vi "SSL Detection Frame Simple Estimator Cameras VelCmd.vi"(0 "Lado":enum16{"Esquerdo", "Direito"}(ring)=enum."Direito" caption="Enum", 4 "Last IA State":T5={"our_robots"=[], "enemy_robots"=[], "balls"=[], "geometry"={"line_width"=0, "field_length"=0, "field_width"=0, "boundary_width"=0, "referee_width"=0, "goal_width"=0, "goal_depth"=0, "goal_wall_width"=0, "center_circle_radius"=0, "defense_radius"=0, "defense_stretch"=0, "free_kick_from_defense_dist"=0, "penalty_spot_from_field_line_dist"=0, "penalty_line_from_spot_dist"=0}, "IA Judge"={"stage"="", "command"="", "our_goalie_id"=0.0, "enemy_goalie_id"=0.0, "command enum"=enum."Halt", "Time"=enum."Azul"}, "Received Timestamp"=timestamp(0 s since 1904-01-01), "Events"={"Touch"=FALSE, "Ball out"=FALSE, "id touch"=0.0, "Ball out of \nVision"=FALSE, "Ball inside \nGoalie area"=FALSE, "Robot not responding"=FALSE, "Robots responding status"=[1.0, 1.0, 1.0, 1.0, 1.0, 1.0], "Enemy Ball \nPossession"=FALSE, "Pass State"=FALSE, "id end of pass"=0.0, "Kick"=FALSE, "Id ini Possession"=0.0, "Ball Possesion"=FALSE, "Id Possesion"=0.0, "Direct Kick"=FALSE, "2nd Strk Ativo"=FALSE}}, 5 "Estimador":T16, 6 "Time":enum16{"Azul", "Amarelo"}(ring) caption="Enum", 7 "Enable":bool, 8 "ignora esquerda?":bool=TRUE, 9 "ignora lado?":bool=TRUE, 10 "Field Size":T17, 11 "Detection Frame":T1 {"robots_blue"."height" format="%+4.3f"; "robots_blue"."pixel_y" format="%+4.3f"; "robots_blue"."pixel_x" format="%+4.3f"; "robots_blue"."orientation" format="%+4.3f"; "robots_blue"."y" format="%+4.3f"; "robots_blue"."confidence" format="%4.3f"; "robots_blue"."x" format="%+4.3f"; "robots_yellow"."height" format="%+4.3f"; "robots_yellow"."pixel_y" format="%+4.3f"; "robots_yellow"."pixel_x" format="%+4.3f"; "robots_yellow"."orientation" format="%+4.3f"; "robots_yellow"."y" format="%+4.3f"; "robots_yellow"."confidence" format="%4.3f"; "robots_yellow"."x" format="%+4.3f"}) -> (2 "Field Size Out":T17, 3 "Detection Frame Out":T1 {"robots_blue"."height" format="%+4.3f"; "robots_blue"."pixel_y" format="%+4.3f"; "robots_blue"."pixel_x" format="%+4.3f"; "robots_blue"."orientation" format="%+4.3f"; "robots_blue"."y" format="%+4.3f"; "robots_blue"."confidence" format="%4.3f"; "robots_blue"."x" format="%+4.3f"; "robots_yellow"."height" format="%+4.3f"; "robots_yellow"."pixel_y" format="%+4.3f"; "robots_yellow"."pixel_x" format="%+4.3f"; "robots_yellow"."orientation" format="%+4.3f"; "robots_yellow"."y" format="%+4.3f"; "robots_yellow"."confidence" format="%4.3f"; "robots_yellow"."x" format="%+4.3f"})   [LabVIEW 2018]
uses:
  SSL Detection Frame.ctl
  SSL Detection Robot.ctl
  <vilib>/Analysis/Matrix/Datatypes/RealMatrix.ctl
  SSL Detection Ball.ctl
  Filters/Estimadores.ctl
  Core/AI Input.ctl
  Core/AI Robot.ctl
  Intel/Functions Enum.ctl
  Intel/AttackerStates.ctl
  Path Planning/RRT/PathDests.ctl
  Path Planning/RRT/PathDest.ctl
  Core/AI Ball.ctl
  Core/Field Size.ctl
  Core/AI Judge.ctl
  Intel/Command Enum.ctl
  Events/Events.ctl
  <vilib>/Analysis/Matrix/NI_Matrix.lvlib
panel:
  out "output cluster":T1 {"robots_blue"."height" format="%+4.3f"; "robots_blue"."pixel_y" format="%+4.3f"; "robots_blue"."pixel_x" format="%+4.3f"; "robots_blue"."orientation" format="%+4.3f"; "robots_blue"."y" format="%+4.3f"; "robots_blue"."confidence" format="%4.3f"; "robots_blue"."x" format="%+4.3f"; "robots_yellow"."height" format="%+4.3f"; "robots_yellow"."pixel_y" format="%+4.3f"; "robots_yellow"."pixel_x" format="%+4.3f"; "robots_yellow"."orientation" format="%+4.3f"; "robots_yellow"."y" format="%+4.3f"; "robots_yellow"."confidence" format="%4.3f"; "robots_yellow"."x" format="%+4.3f"}
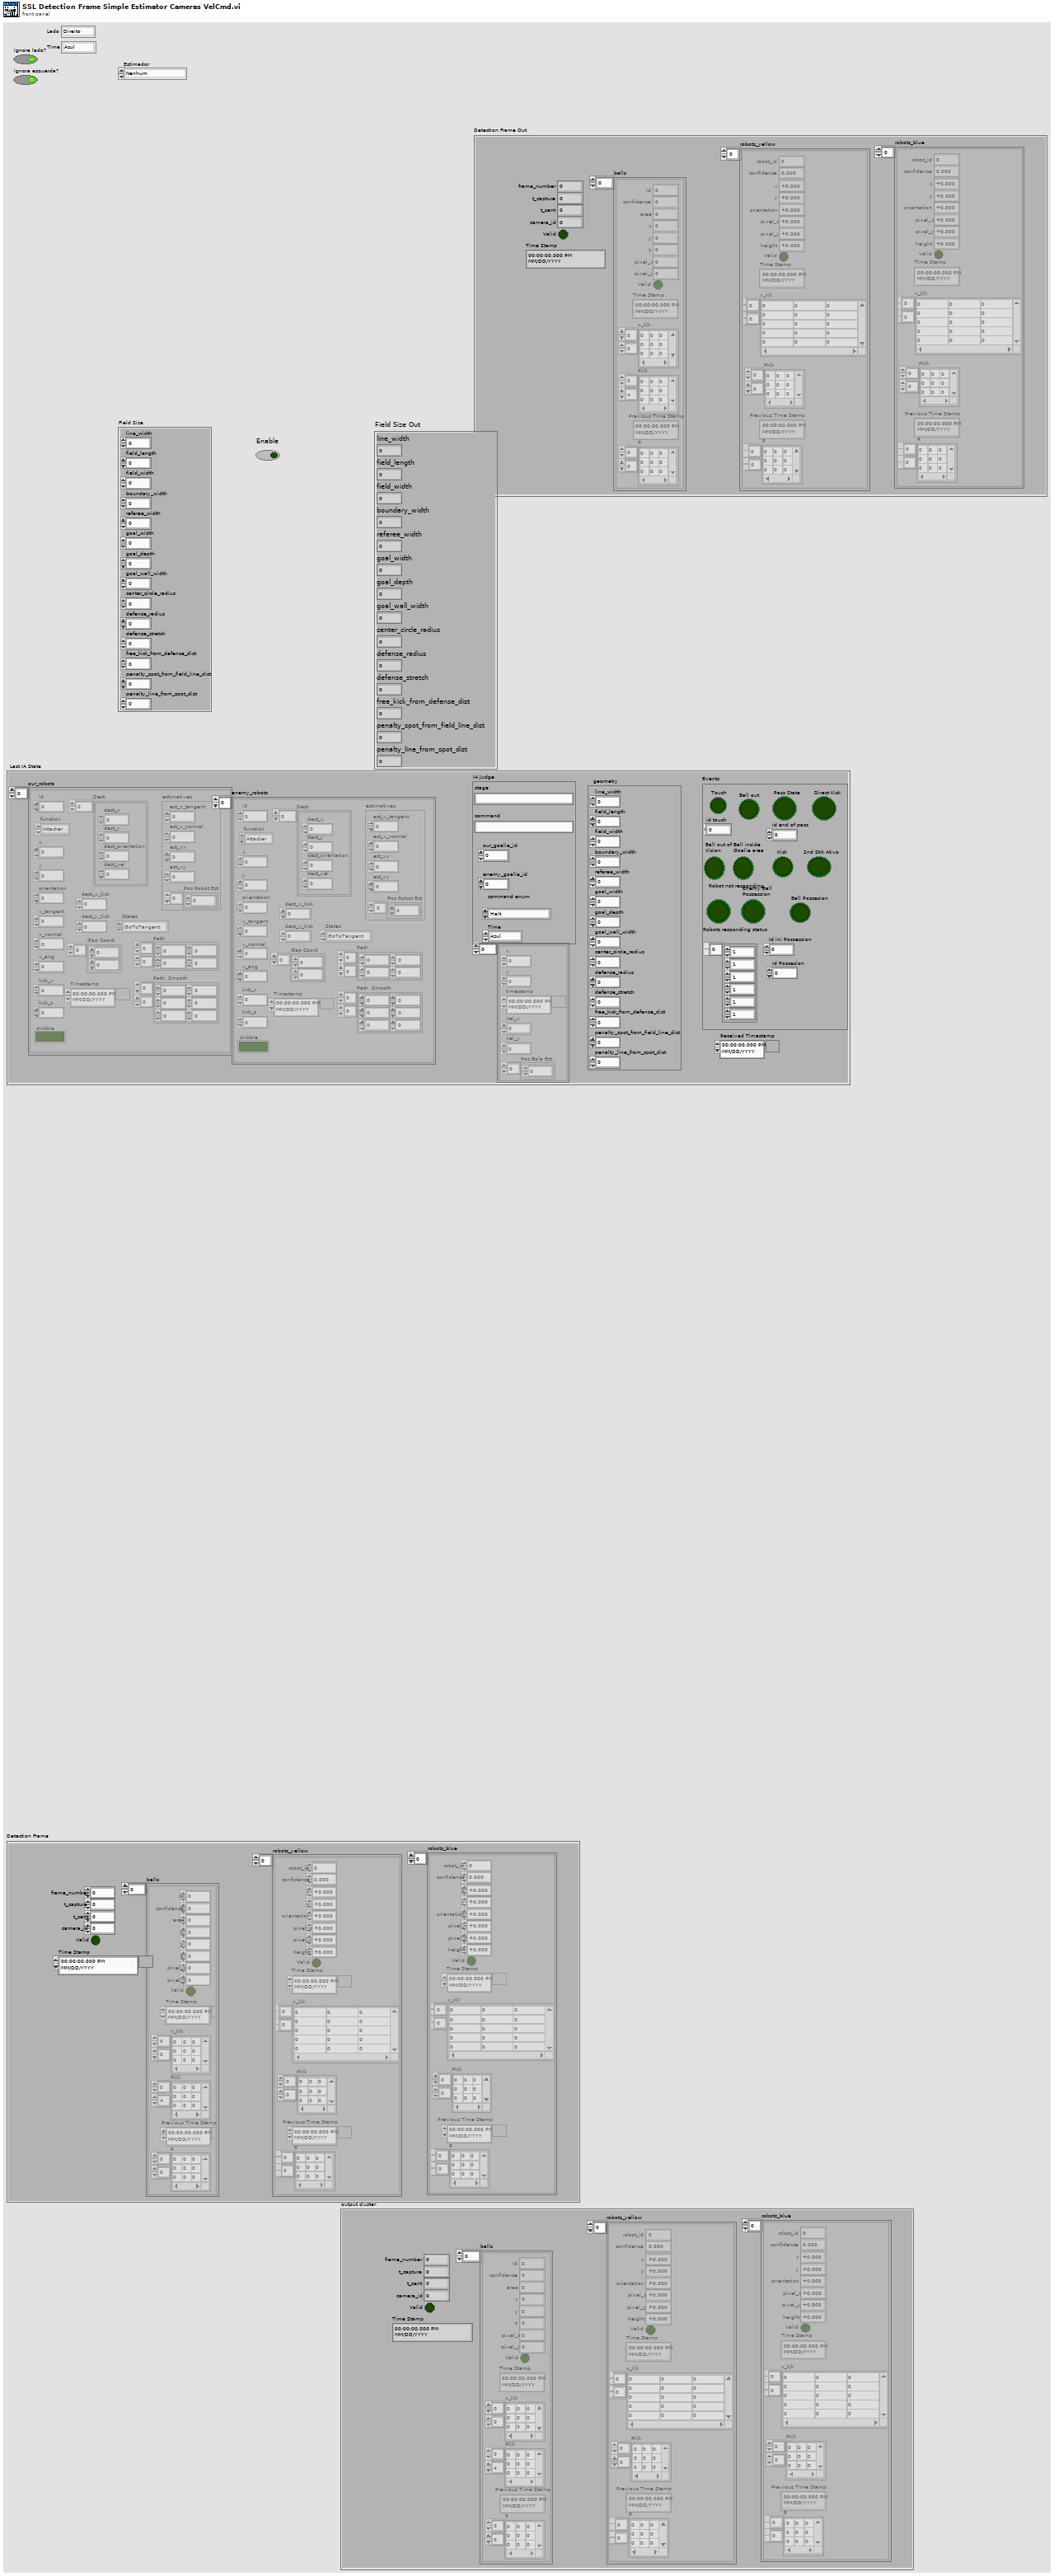
[diagram p1: front panel]
types:
  T1 = typedef "SSL Detection Frame.ctl" = cluster{"frame_number":u32, "t_capture":dbl, "t_sent":dbl, "camera_id":u32, "robots_yellow":T2[], "robots_blue":T2[], "balls":T4[], "Valid":bool, "Time Stamp":timestamp}
  T2 = typedef "SSL Detection Robot.ctl" = cluster{"x":sgl, "robot_id":u32, "confidence":sgl, "y":sgl, "orientation":sgl, "pixel_x":sgl, "pixel_y":sgl, "height":sgl, "Valid":bool, "Time Stamp":timestamp, "x_k|k":T3, "Pk|k":T3, "Previous Time Stamp":timestamp, "R":T3}
  T3 = typedef "NI_Matrix.lvlib/RealMatrix.ctl" = dbl[][]
  T4 = typedef "SSL Detection Ball.ctl" = cluster{"x":sgl, "area":u32, "confidence":sgl, "y":sgl, "z":sgl, "pixel_x":sgl, "pixel_y":sgl, "Valid":bool, "Time Stamp":timestamp, "x_k|k":T3, "Pk|k":T3, "Id":u32, "Previous Time Stamp":timestamp, "R":T3}
  T5 = typedef "AI Input.ctl" = cluster{"our_robots":T6[], "enemy_robots":T6[], "balls":T11[], "geometry":T12, "IA Judge":T13, "Received Timestamp":timestamp, "Events":T15}
  T6 = typedef "AI Robot.ctl" = cluster{"id":u32, "function":T7, "x":dbl, "y":dbl, "orientation":dbl, "v_tangent":dbl, "v_normal":dbl, "v_ang":dbl, "kick_x":dbl, "kick_z":dbl, "dribble":bool, "Timestamp":timestamp, "estimatives":cluster{"est_v_tangent":dbl, "est_v_normal":dbl, "est_vx":dbl, "est_vy":dbl, "Pos Robot Est":dbl[]}, "dest_x_kick":dbl, "dest_y_kick":dbl, "Gap Coord":dbl[], "States":T8, "Path ":dbl[][], "Path  Smooth":dbl[][], "Dest":T9}
  T7 = typedef "Functions Enum.ctl" = enum16{"2nd Striker", "Attacker", "Goalie", "Defender", "Striker", "Goto 0", "Dummy", "Kicker", "ZigZag 0", "ZigZag 1", "ZigZag 2", "ZigZag 3", "ZigZag 4", "ZigZag 5", "ZigZag 6", "ZigZag 7", "ZigZag 8", ""}
  T8 = typedef "AttackerStates.ctl" = enum16{"Pass", "GoToTangent", "BallGetting", "GoToKick", ""}
  T9 = typedef "PathDests.ctl" = T10[]
  T10 = typedef "PathDest.ctl" = cluster{"dest_x":dbl, "dest_y":dbl, "dest_orientation":dbl, "dest_vel":dbl}
  T11 = typedef "AI Ball.ctl" = cluster{"x":dbl, "y":dbl, "timestamp":timestamp, "Vel_x":dbl, "Vel_y":dbl, "Pos Bola Est":dbl[]}
  T12 = typedef "Field Size.ctl" = cluster{"line_width":u32, "field_length":u32, "field_width":u32, "boundary_width":u32, "referee_width":u32, "goal_width":u32, "goal_depth":u32, "goal_wall_width":u32, "center_circle_radius":u32, "defense_radius":u32, "defense_stretch":u32, "free_kick_from_defense_dist":u32, "penalty_spot_from_field_line_dist":u32, "penalty_line_from_spot_dist":u32}
  T13 = typedef "AI Judge.ctl" = cluster{"stage":string, "command":string, "our_goalie_id":dbl, "enemy_goalie_id":dbl, "command enum":T14, "Time":enum16{"Azul", "Amarelo"}}
  T14 = typedef "Command Enum.ctl" = enum16{"Halt", "Stop", "Force Start", "PKA Normal Start", "Prepare Kickoff Ally", "PKE Normal Start", "Prepare Kickoff Enemy", "Prepare Penalty Ally", "PPA Normal Start", "Prepare Penalty Enemy", "PPE Normal Start", "Direct Free Enemy", "Direct Free Ally", "Indirect Free Enemy", "Indirect Free Ally", "Timeout Enemy", "Timeout Ally", "Goal Enemy", "Goal Ally", "Ball Placement Enemy", "Ball Placement Ally", "Normal Half Time", "Extra Time Break", "Extra Half Time", "None", "Post Game"}
  T15 = typedef "Events.ctl" = cluster{"Touch":bool, "Ball out":bool, "id touch":dbl, "Ball out of \nVision":bool, "Ball inside \nGoalie area":bool, "Robot not responding":bool, "Robots responding status":dbl[], "Enemy Ball \nPossession":bool, "Pass State":bool, "id end of pass":dbl, "Kick":bool, "Id ini Possession":dbl, "Ball Possesion":bool, "Id Possesion":dbl, "Direct Kick":bool, "2nd Strk Ativo":bool}
  T16 = typedef "Estimadores.ctl" = enum16{"Nenhum", "Simples", "Kalman"}
  T17 = cluster{"line_width":u32, "field_length":u32, "field_width":u32, "boundary_width":u32, "referee_width":u32, "goal_width":u32, "goal_depth":u32, "goal_wall_width":u32, "center_circle_radius":u32, "defense_radius":u32, "defense_stretch":u32, "free_kick_from_defense_dist":u32, "penalty_spot_from_field_line_dist":u32, "penalty_line_from_spot_dist":u32}
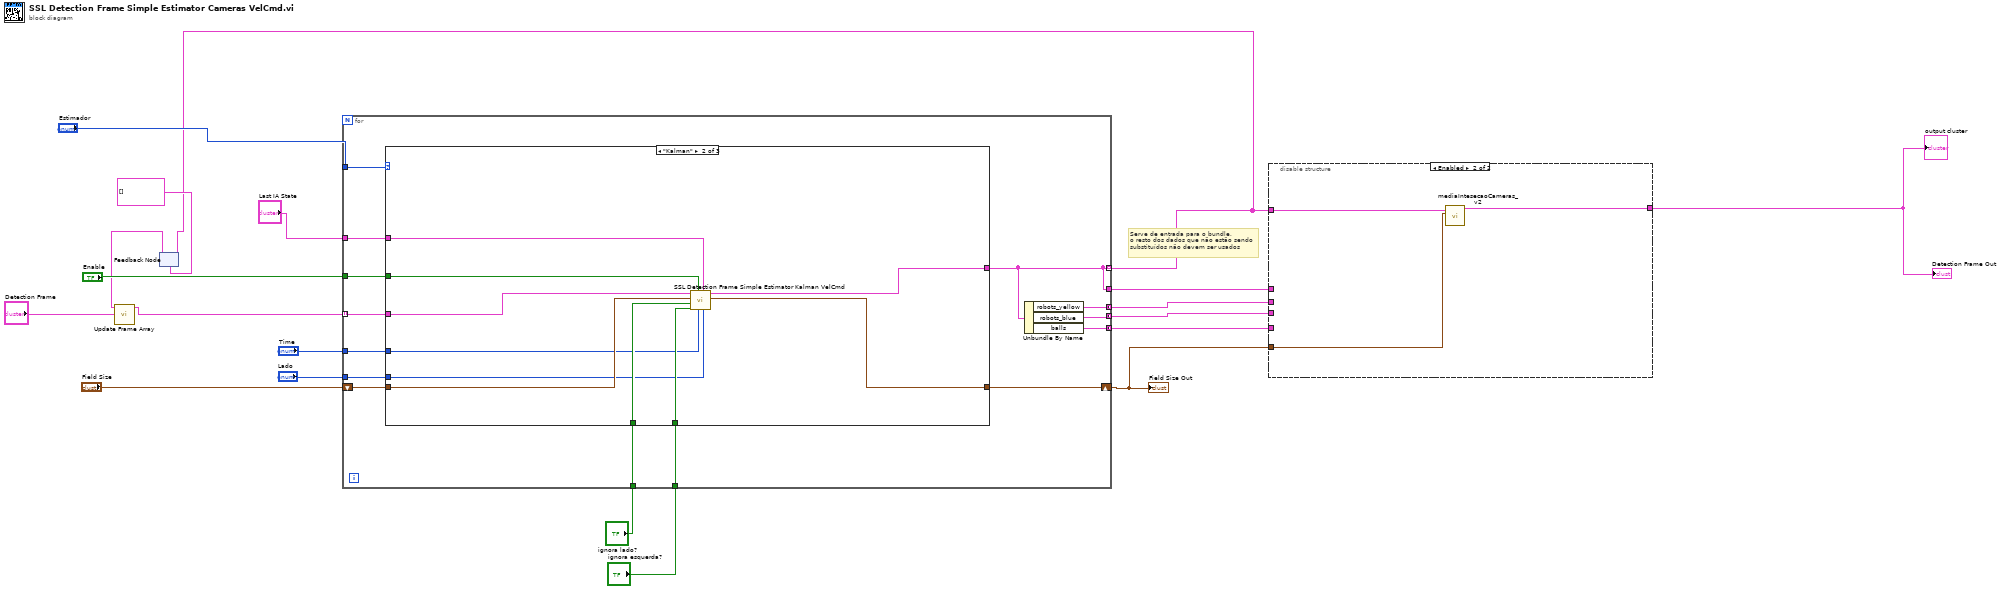
[diagram p0: block diagram]
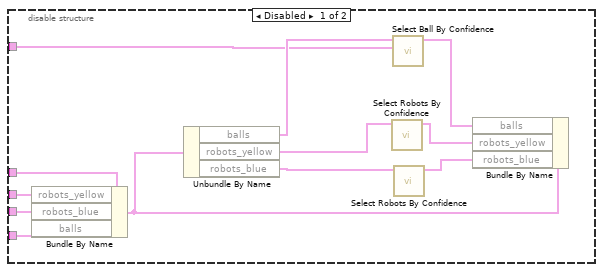
[diagram p2: hidden frame]
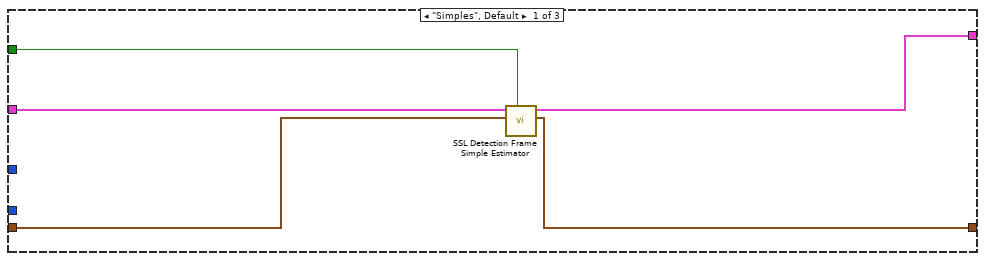
[diagram p3: hidden frame]
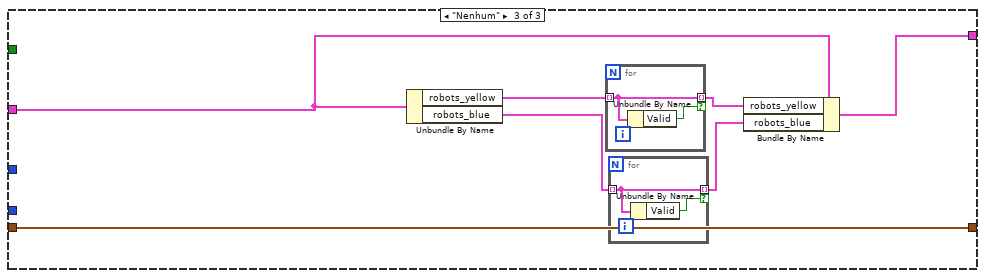
[diagram p4: hidden frame]
diagram:
  # "Serve de entrada para o bundle, \no resto dos dados que não estão sendo\nsubstituídos não devem ser usados"
  n1 = feedback #1(T1[] []) -> (w5:T1[])
  n2 = call "Update Frame Array.vi"("Detection Frame In"="Detection Frame", "Array Detection Frame In"=w5) -> ("Detection Frame In out"=w7:T1[])  [unwired: 9 in]
  n3 = for {
    tunnel: [w25] -> w2 mode=indexing
    tunnel: "Estimador" -> [w31]
    tunnel: "Enable" -> [w30]
    tunnel: w7 -> [w29] mode=indexing
    shift-right: [w32] -> w1
    shift-left: "Field Size" -> [w33]
    tunnel: [w28] -> w17 mode=concatenating
    tunnel: [w27] -> w16 mode=concatenating
    tunnel: [w26] -> w12 mode=concatenating
    tunnel: [w25] -> w18
    tunnel: "ignora lado?" -> [w24]
    tunnel: "ignora esquerda?" -> [w23]
    tunnel: "Time" -> [w22]
    tunnel: "Last IA State" -> [w21]
    tunnel: "Lado" -> [w20]
    n4 = case shown="\"Kalman\"" w31 {
      tunnel: [w34 w47 w51] -> w25
      tunnel: w29 -> [w38 w48 w53]
      tunnel: w30 -> [w37 w44 _]
      tunnel: w33 -> [w36 w46 w55]
      tunnel: [w35 w45 w55] -> w32
      tunnel: w24 -> [_ w43 _]
      tunnel: w23 -> [_ w42 _]
      tunnel: w22 -> [_ w41 _]
      tunnel: w21 -> [_ w40 _]
      tunnel: w20 -> [_ w39 _]
      frame "Simples", Default {
        n5 = call "SSL Detection Frame Simple Estimator.vi"("Enable"=w37, "Field Size"=w36, "Detection Frame In"=w38) -> ("Field Size Out"=w35:T17, "Detection Frame Out"=w34:T1)  [unwired: 7 in]
      }
      frame "Kalman" {
        n6 = call "SSL Detection Frame Simple Estimator Kalman VelCmd.vi"("Lado"=w39, "Last IA State"=w40, "Time"=w41, "Enable"=w44, "ignora esquerda?"=w42, "ignora lado?"=w43, "Field Size"=w46, "Detection Frame In"=w48) -> ("Field Size Out"=w45:T17, "Detection Frame Out"=w47:T1)  [unwired: 2 in]
      }
      frame "Nenhum" {
        n7 = Unbundle By Name(w53) -> ("robots_yellow"=w54:T2[], "robots_blue"=w50:T2[])
        n8 = for {
          tunnel: w54 -> [w59] mode=indexing
          tunnel: [w59] -> w52 mode=indexing if=w58
          n9 = Unbundle By Name(w59) -> ("Valid"=w58:bool)
        }
        n10 = for {
          tunnel: w50 -> [w57] mode=indexing
          tunnel: [w57] -> w49 mode=indexing if=w56
          n11 = Unbundle By Name(w57) -> ("Valid"=w56:bool)
        }
        n12 = Bundle By Name(cluster=w53, "robots_yellow"=w52, "robots_blue"=w49) -> (w51:T1)
      }
    }
    n13 = Unbundle By Name(w25) -> ("robots_yellow"=w28:T2[], "robots_blue"=w27:T2[], "balls"=w26:T4[])
  }
  "Field Size Out" <- w1
  n14 = feedback-in #1(w2) -> ()
  n15 = disable-structure shown="Enabled" {
    disable-tunnel: w18 -> [w72 _]
    disable-tunnel: w17 -> [w71 _]
    disable-tunnel: w16 -> [w70 _]
    disable-tunnel: w12 -> [w65 _]
    disable-tunnel: w2 -> [w62 w75]
    disable-tunnel: [_ w74] -> w3
    disable-tunnel: w1 -> [_ w73]
    frame Disabled {
      n16 = Bundle By Name(cluster=w72, "robots_yellow"=w71, "robots_blue"=w70, "balls"=w65) -> (w61:T1)
      n17 = Unbundle By Name(w61) -> ("balls"=w64:T4[], "robots_yellow"=w67:T2[], "robots_blue"=w69:T2[])
      n18 = call "Select Robots By Confidence.vi"("robots_blue"=w67) -> ("Array"=w66:T2[])  [unwired: 10 in]
      n19 = call "Select Ball By Confidence.vi"("Array"=w62, "balls"=w64) -> ("balls out"=w63:T4[])  [unwired: 9 in]
      n20 = call "Select Robots By Confidence.vi"("robots_blue"=w69) -> ("Array"=w68:T2[])  [unwired: 10 in]
      n21 = Bundle By Name(cluster=w61, "balls"=w63, "robots_yellow"=w66, "robots_blue"=w68) -> (w60:T1)
    }
    frame Enabled {
      n22 = call "mediaIntesecaoCameras_v2.vi"("Field Geometry In"=w73, "Cameras Array"=w75) -> ("frame out"=w74:T1)  [unwired: 9 in]
    }
  }
  "Detection Frame Out" <- w3
  "output cluster" <- w3
